vi "getClassInfo.vi"(0 "reference in":refnum<class "VINode.lvclass">, 5 "error in (no error)":errorcluster) -> (9 "ModuleUnmodified":path, 12 "Base class.bounds":T1 {"height" format="%.2f"; "width" format="%.2f"; "y" format="%.2f"; "x" format="%.2f"}, 14 "reference out":refnum<class "VINode.lvclass">, 15 "className":string, 18 "ModulePath":path, 19 "error out":errorcluster)   [LabVIEW 2014, in "VINode.lvclass"]
uses:
  <resource>/Framework/Providers/Open_GDS/UML/VINode_class/VINode.lvclass
  <resource>/Framework/Providers/Open_GDS/UML/General/Rectangle/Rectangle Rectangle2D.ctl
  <resource>/Framework/Providers/Open_GDS/UML/MultiLineString_class/MultiLineString.lvclass
  <resource>/Framework/Providers/Open_GDS/UML/RectangularNode_class/RectangularNode.lvclass
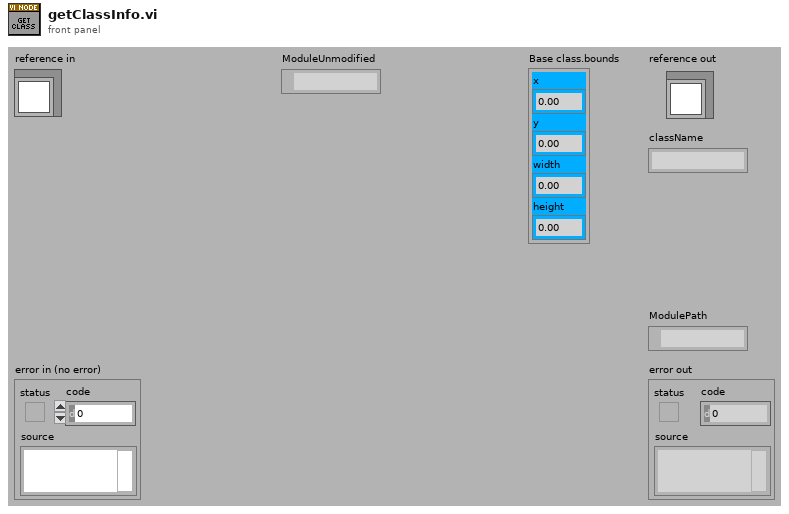
[diagram p1: front panel]
types:
  T1 = typedef "Rectangle Rectangle2D.ctl" = cluster{"x":dbl, "y":dbl, "width":dbl, "height":dbl}
  T2 = typedef "VINode.lvclass/ObjectAttributes.ctl" = cluster{"midHeight":dbl, "botHeight":dbl, "Name":refnum<class "MultiLineString.lvclass">, "DEFAULT_COMPARTMENT_HEIGHT":i32, "DEFAULT_WIDTH":i32, "DEFAULT_HEIGHT":i32, "VIPath":path, "Description":refnum<class "MultiLineString.lvclass">, "ShowDescription":bool}
  T3 = typedef "RectangularNode.lvclass/ObjectAttributes.ctl" = cluster{"bounds":T1}
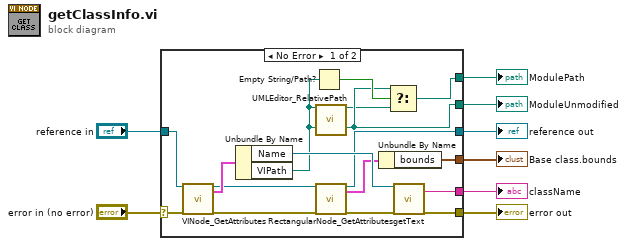
[diagram p0: block diagram]
diagram:
  n1 = case shown="No Error" "error in (no error)" {
    selector: "error in (no error)" -> [w24 w25]
    tunnel: "reference in" -> [w23 w26]
    tunnel: [w10 w25] -> w6
    tunnel: [w12 w26] -> w5
    tunnel: [w21 _] -> w4
    tunnel: [w17 _] -> w3
    tunnel: [w19 _] -> w2
    tunnel: [w16 _] -> w1
    frame No Error {
      n2 = call <resource>:"VINode_GetAttributes.vi"("reference in"=w23, "error in (no error)"=w24) -> ("reference out"=w14:refnum<class "VINode.lvclass">, "Data"=w15:T2, "error out"=w13:errorcluster)  [unwired: 1 in, 14 out]
      n3 = Unbundle By Name(w15) -> ("Name"=w22:refnum<class "MultiLineString.lvclass">, "VIPath"=w19:path)
      n4 = Empty String/Path?(string/path=w19) -> (empty?=w20:bool)
      n5 = call <resource>:"UMLEditor_RelativePath.vi"("Path In"=w19) -> ("ConvertToAbsolutePath(If possible)"=w18:path)  [unwired: 1 in, 17 out]
      n6 = call <resource>:"RectangularNode_GetAttributes.vi"("reference in"=w14, "error in (no error)"=w13) -> ("reference out"=w12:refnum<class "VINode.lvclass">, "Data"=w11:T3, "error out"=w9:errorcluster)  [unwired: 14 in, 1 out]
      n7 = Unbundle By Name(w11) -> ("bounds"=w16:T1)
      n8 = Select(t=w19, s=w20, f=w18) -> (s? t:f=w17:path)
      n9 = call-dynamic "getText.vi"("reference"=w22, "error in (no error)"=w9) -> ("text"=w21:string, "error out"=w10:errorcluster)  [unwired: 16 out]
    }
    frame Error {
    }
  }
  "reference out" <- w5
  "error out" <- w6
  "className" <- w4
  "ModulePath" <- w3
  "ModuleUnmodified" <- w2
  "Base class.bounds" <- w1
